vi "pulmonarytesting.vi"() -> ()   [LabVIEW 2014]
uses:
  <vilib>/vision/NI_Vision_Development_Module.lvlib
  <instrlib>/KD Scientific 2XX Series/KD Scientific 2XX Series.lvlib
panel:
  in  "Baud Rate (9600)":u32(ring)=9600 items=["300"=300, "1200"=1200, "2400"=2400, "4800"=4800, "9600"=9600]
  in  "Withdrawal Settings":T1={"Flow Rate (5)"=5.0, "Volume (10)"=10.0, "Volume Units (ml)"=enum."milliliters (ml)", "Rate Units (ml/min.)"=enum."milliliters per minute (ml/min.)"} {"Volume (10)" format="%#.3g"}
  in  "Diameter (8.75 mm)":dbl=8.75
  in  "Infusion Settings":T1={"Flow Rate (5)"=5.0, "Volume (10)"=10.0, "Volume Units (ml)"=enum."milliliters (ml)", "Rate Units (ml/min.)"=enum."milliliters per minute (ml/min.)"}
  out "Status":T2
  in  "stop 2":bool
  out "Delivered Volume":dbl
  out "Units":string
  in  "Operation Mode (Infuse)":u16(ring) items=["Infuse", "Withdraw", "Infuse-Withdraw", "Withdraw-Infuse", "Continuous"]
  in  "Address (0)":i32 format="%0.0f"
  in  "error in (no error)":errorcluster
  in  "VISA resource name":refnum<visa-resource-name>="COM1"
  in  "stop":bool
  out "Image":T3(plugin-control)
  out "Particle Measurements (Pixels) (Particle Analysis 1)":dbl[][](array[numeric]) format="%.2f"
  out "subarray":dbl[](array[numeric])
  out "The diameter":dbl[](array[numeric])
  out "Image from  Vision Acquisition 1":T3(plugin-control)
  in  "stop (F)":bool
  out "Data from Transducer":dynamicdata(graph) caption="Voltage from Transducer V"
  out "Voltage from pressure transducer":dbl[](array[numeric])
  out "Pressure mm Hg":dbl[](graph)
  in  "Calibration factor":dbl[](array[numeric])
  in  "Zero Error":dbl[](array[numeric])
  out "pressure mm Hg":dbl[](array[numeric])
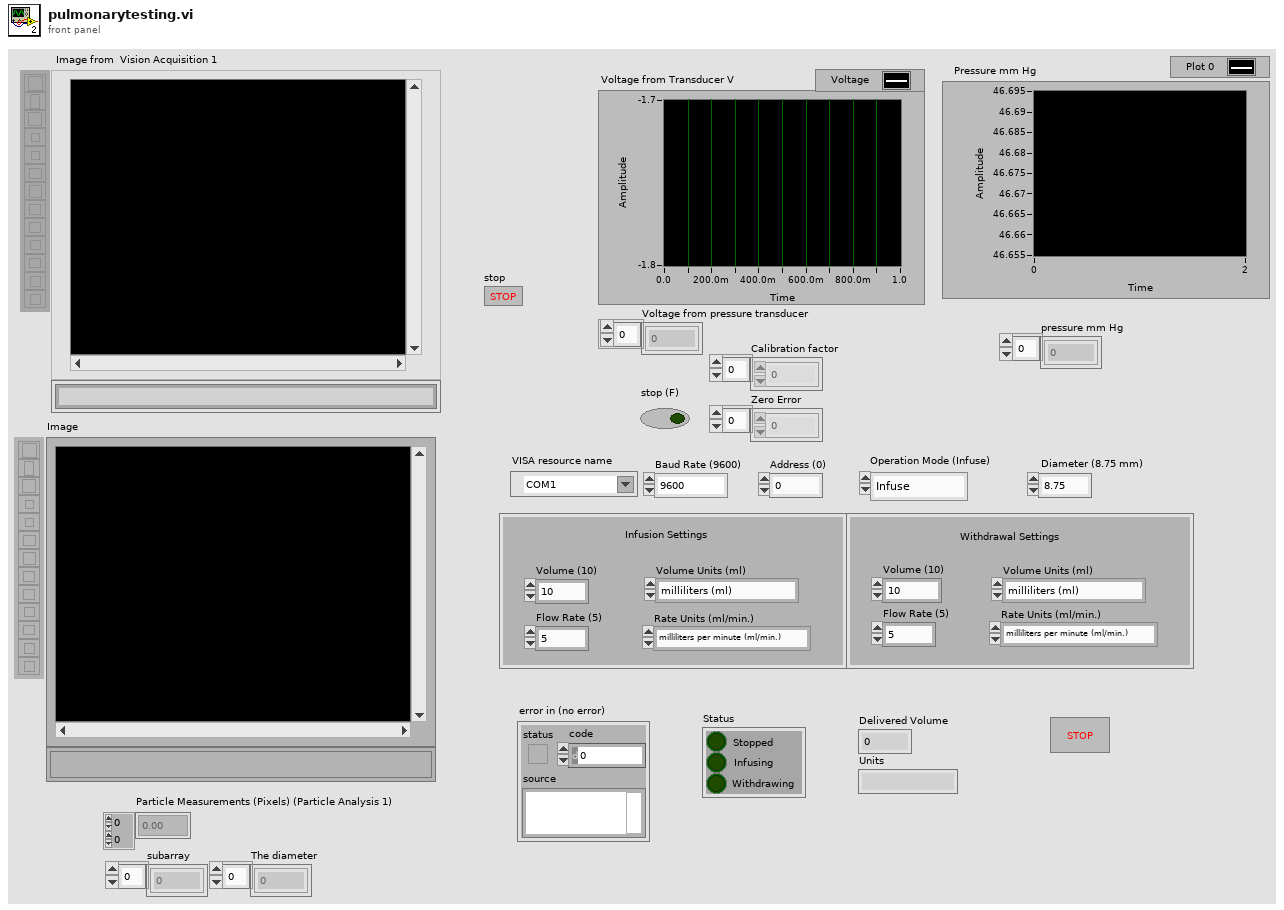
[diagram p1: front panel]
types:
  T1 = cluster{"Flow Rate (5)":dbl, "Volume (10)":dbl, "Volume Units (ml)":enum16{"milliliters (ml)", "microliters (ul)"}, "Rate Units (ml/min.)":enum16{"milliliters per minute (ml/min.)", "milliliters per hour (ml/hr.)", "microliters per minute (ul/min.)", "microliters per hour (ul/hr.)"}}
  T2 = cluster{"Stopped":bool, "Infusing":bool, "Withdrawing":bool}
  T3 = typedef "IMAQ Image.ctl" = refnum<image>
  T4 = typedef "Board Id" = u8
  T5 = typedef "ROI Descriptor" = cluster{"Global Rectangle":i32[], "Contours":cluster{"ID":enum32{"External", "Internal"}, "Type":u32, "Coordinates":i32[]}[]}
  T6 = enum16{"milliliters per minute (ml/min.)", "milliliters per hour (ml/hr.)", "microliters per minute (ul/min.)", "microliters per hour (ul/hr.)"}
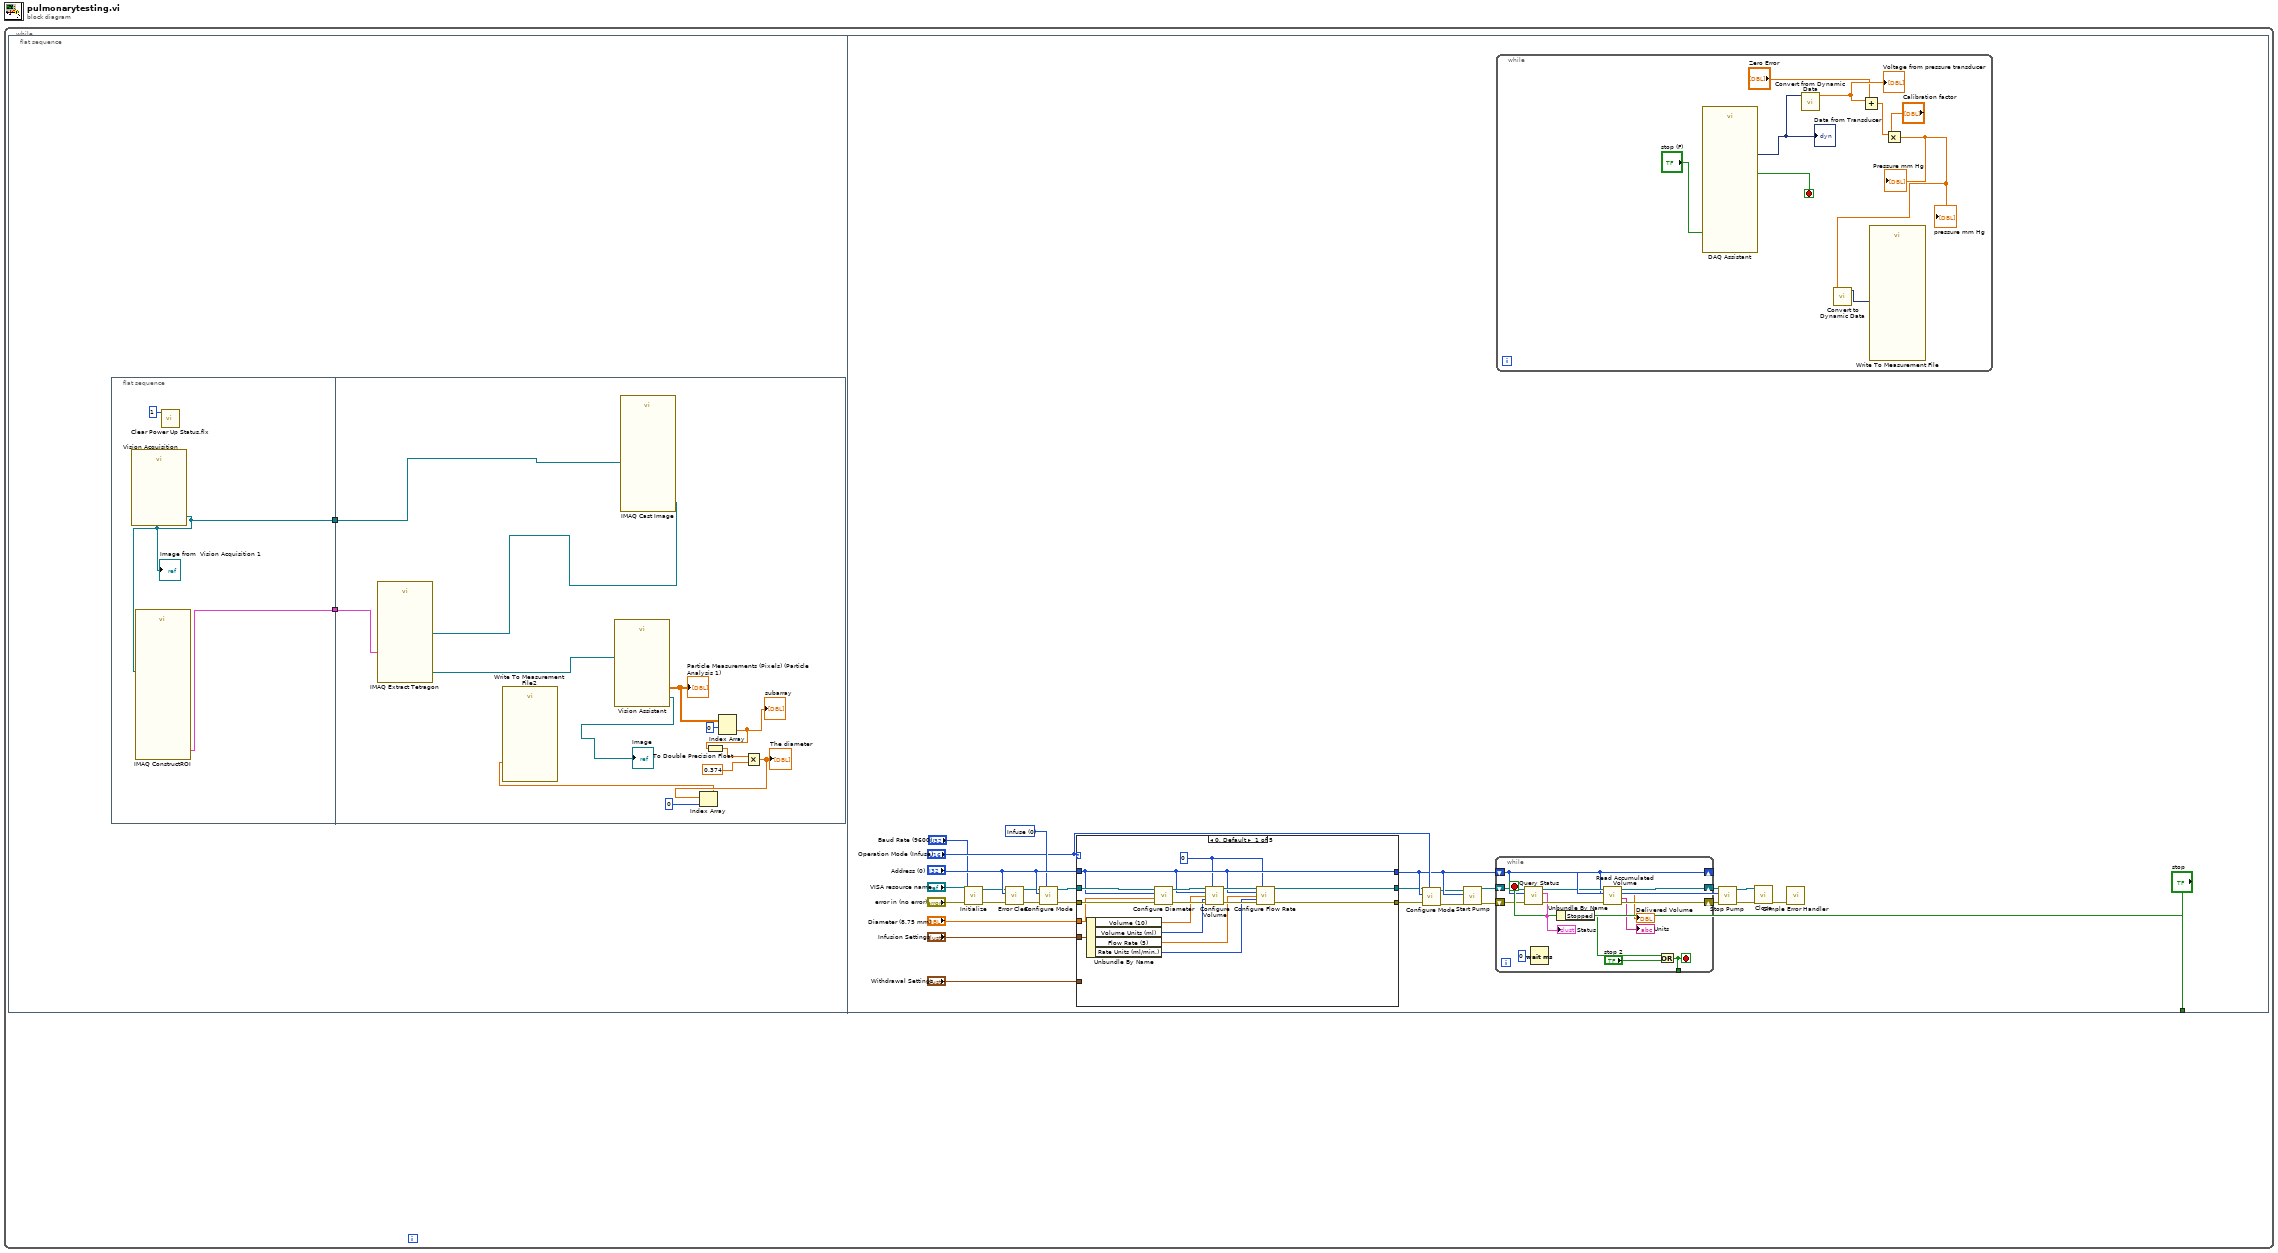
[diagram p0: block diagram]
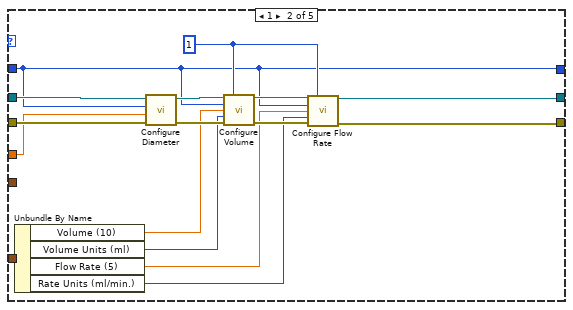
[diagram p2: hidden frame]
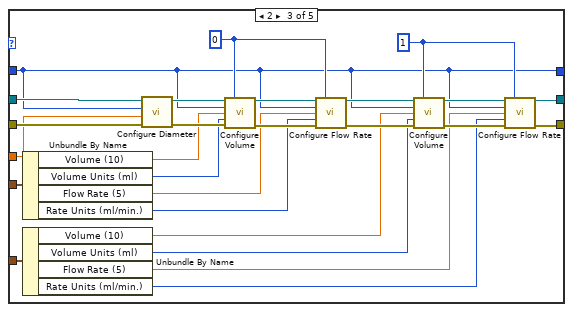
[diagram p3: hidden frame]
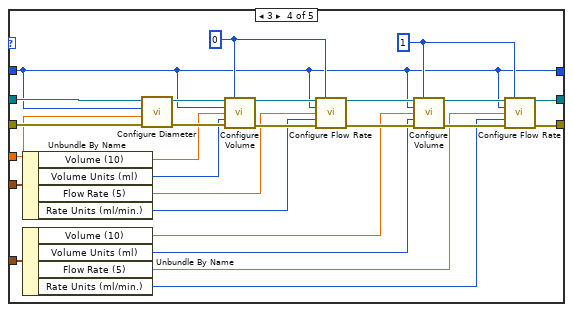
[diagram p4: hidden frame]
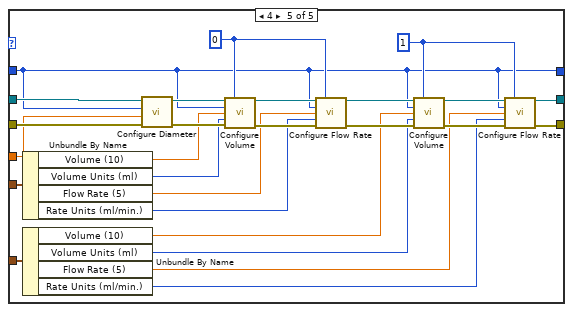
[diagram p5: hidden frame]
diagram:
  n1 = while {
    stop <- w1 stop-if-true
    n2 = flat-sequence {
      tunnel: ["stop"] -> w1
      frame #0 {
        n3 = flat-sequence {
          tunnel: [w6] -> w3
          tunnel: [w4] -> w2
          tunnel: w3 -> [w19]
          tunnel: w2 -> [w10]
          frame #0 {
            n4 = call "Vision Acquisition"() -> ("Image Out"=w4:T3)  [unwired: 25 in, 2 out]
            "Image from  Vision Acquisition 1" <- w4
            n5 = call "IMAQ ConstructROI"("Image"=w4) -> ("ROI Descriptor Out"=w6:T5)  [unwired: 7 in, 3 out]
            n6 = call <vilib>:"Clear Power Up Status.flx"("Board ID"=T4 1) -> ()  [unwired: 6 in, 2 out]
          }
          frame #1 {
            n7 = call "IMAQ Cast Image"("Image Src"=w10) -> ("Image Dst Out"=w16:T3)  [unwired: 9 in, 1 out]
            n8 = call-poly "IMAQ Extract Tetragon"("ROI Descriptor"=w19, "Image Src"=w16) -> ("Image Dst Out"=w17:T3)  [unwired: 8 in, 1 out]
            n9 = call "Vision Assistant"("Image In"=w17) -> ("Image Out"=→"Image":T3, "Particle Measurements (Pixels) (Particle Analysis 1)"=w15:dbl[][])  [unwired: 23 in, 2 out]
            "Particle Measurements (Pixels) (Particle Analysis 1)" <- w15
            n10 = Index Array(array=w15, index (row)=0) -> (element=w13:dbl[])  [unwired: 1 in]
            "subarray" <- w13
            n11 = To Double Precision Float(number=w13) -> (double precision float=w12:dbl[])
            n12 = Multiply(x=w12, y=0.374) -> (x*y=w9:dbl[])
            "The diameter" <- w9
            n13 = Index Array(array=w9, index=0) -> (element=w7:dbl)
            n14 = call "Write To Measurement File2"("Signals"=w7) -> ()  [unwired: 16 in, 3 out]
          }
        }
      }
      frame #1 {
        w42 = u16 0 items=["Infuse", "Withdraw", "Infuse-Withdraw", "Withdraw-Infuse", "Continuous"] ("Mode (infuse)")
        n15 = call <instrlib>:"Initialize.vi"("error in (no error)"="error in (no error)", "Baud Rate (9600)"="Baud Rate (9600)", "VISA resource name"="VISA resource name") -> ("error out"=w45:errorcluster, "VISA resource name out"=w46:refnum<visa-resource-name>)  [unwired: 7 in]
        n16 = call <instrlib>:"Error Clear.vi"("error in (no error)"=w45, "Address (0)"="Address (0)", "VISA resource name"=w46) -> ("error out"=w44:errorcluster, "VISA resource name out"=w43:refnum<visa-resource-name>)  [unwired: 6 in, 1 out]
        n17 = call <instrlib>:"Configure Mode.vi"("Mode (infuse)"=w42, "error in (no error)"=w44, "Address (0)"="Address (0)", "VISA resource name"=w43) -> ("error out"=w40:errorcluster, "VISA resource name out"=w41:refnum<visa-resource-name>)  [unwired: 6 in]
        n18 = case shown="0, Default" "Operation Mode (Infuse)" {
          tunnel: "Infusion Settings" -> [w58 _ w106 w132 w158]
          tunnel: "Withdrawal Settings" -> [_ w80 w105 w131 w157]
          tunnel: w41 -> [w64 w79 w104 w130 w156]
          tunnel: w40 -> [w63 w75 w103 w129 w155]
          tunnel: "Diameter (8.75 mm)" -> [w57 w71 w86 w112 w138]
          tunnel: [w56 w65 w81 w107 w133] -> w38
          tunnel: "Address (0)" -> [w56 w65 w81 w107 w133]
          tunnel: [w51 w76 w83 w109 w135] -> w34
          tunnel: [w50 w72 w82 w108 w134] -> w35
          frame 0, Default {
            w49 = 0
            n19 = Unbundle By Name(w58) -> ("Volume (10)"=w55:dbl, "Volume Units (ml)"=w54:enum16{"milliliters (ml)", "microliters (ul)"}, "Flow Rate (5)"=w53:dbl, "Rate Units (ml/min.)"=w52:T6)
            n20 = call <instrlib>:"Configure Diameter.vi"("error in (no error)"=w63, "Diameter (8.75 mm)"=w57, "Address (0)"=w56, "VISA resource name"=w64) -> ("error out"=w61:errorcluster, "VISA resource name out"=w62:refnum<visa-resource-name>)  [unwired: 6 in]
            n21 = call <instrlib>:"Configure Volume.vi"("VISA resource name"=w62, "Mode (infuse)"=w49, "Address (0)"=w56, "Volume (100)"=w55, "Units (0: milliliters)"=w54, "error in (no error)"=w61) -> ("VISA resource name out"=w60:refnum<visa-resource-name>, "error out"=w59:errorcluster)  [unwired: 8 in]
            n22 = call <instrlib>:"Configure Flow Rate.vi"("VISA resource name"=w60, "Mode (infuse)"=w49, "Address (0)"=w56, "Flow Rate (5)"=w53, "Units (0: milliliters per minute)"=w52, "error in (no error)"=w59) -> ("VISA resource name out"=w51:refnum<visa-resource-name>, "error out"=w50:errorcluster)  [unwired: 8 in]
          }
          frame 1 {
            w66 = 1
            n23 = Unbundle By Name(w80) -> ("Volume (10)"=w70:dbl, "Volume Units (ml)"=w69:enum16{"milliliters (ml)", "microliters (ul)"}, "Flow Rate (5)"=w68:dbl, "Rate Units (ml/min.)"=w67:T6)
            n24 = call <instrlib>:"Configure Diameter.vi"("error in (no error)"=w75, "Diameter (8.75 mm)"=w71, "Address (0)"=w65, "VISA resource name"=w79) -> ("error out"=w74:errorcluster, "VISA resource name out"=w78:refnum<visa-resource-name>)  [unwired: 6 in]
            n25 = call <instrlib>:"Configure Volume.vi"("VISA resource name"=w78, "Mode (infuse)"=w66, "Address (0)"=w65, "Volume (100)"=w70, "Units (0: milliliters)"=w69, "error in (no error)"=w74) -> ("VISA resource name out"=w77:refnum<visa-resource-name>, "error out"=w73:errorcluster)  [unwired: 8 in]
            n26 = call <instrlib>:"Configure Flow Rate.vi"("VISA resource name"=w77, "Mode (infuse)"=w66, "Address (0)"=w65, "Flow Rate (5)"=w68, "Units (0: milliliters per minute)"=w67, "error in (no error)"=w73) -> ("VISA resource name out"=w76:refnum<visa-resource-name>, "error out"=w72:errorcluster)  [unwired: 8 in]
          }
          frame 2 {
            w84 = 1
            w85 = 0
            n27 = Unbundle By Name(w106) -> ("Volume (10)"=w94:dbl, "Volume Units (ml)"=w93:enum16{"milliliters (ml)", "microliters (ul)"}, "Flow Rate (5)"=w92:dbl, "Rate Units (ml/min.)"=w91:T6)
            n28 = Unbundle By Name(w105) -> ("Volume (10)"=w90:dbl, "Volume Units (ml)"=w89:enum16{"milliliters (ml)", "microliters (ul)"}, "Flow Rate (5)"=w88:dbl, "Rate Units (ml/min.)"=w87:T6)
            n29 = call <instrlib>:"Configure Diameter.vi"("error in (no error)"=w103, "Diameter (8.75 mm)"=w86, "Address (0)"=w81, "VISA resource name"=w104) -> ("error out"=w98:errorcluster, "VISA resource name out"=w102:refnum<visa-resource-name>)  [unwired: 6 in]
            n30 = call <instrlib>:"Configure Volume.vi"("VISA resource name"=w102, "Mode (infuse)"=w85, "Address (0)"=w81, "Volume (100)"=w94, "Units (0: milliliters)"=w93, "error in (no error)"=w98) -> ("VISA resource name out"=w101:refnum<visa-resource-name>, "error out"=w97:errorcluster)  [unwired: 8 in]
            n31 = call <instrlib>:"Configure Flow Rate.vi"("VISA resource name"=w101, "Mode (infuse)"=w85, "Address (0)"=w81, "Flow Rate (5)"=w92, "Units (0: milliliters per minute)"=w91, "error in (no error)"=w97) -> ("VISA resource name out"=w100:refnum<visa-resource-name>, "error out"=w96:errorcluster)  [unwired: 8 in]
            n32 = call <instrlib>:"Configure Volume.vi"("VISA resource name"=w100, "Mode (infuse)"=w84, "Address (0)"=w81, "Volume (100)"=w90, "Units (0: milliliters)"=w89, "error in (no error)"=w96) -> ("VISA resource name out"=w99:refnum<visa-resource-name>, "error out"=w95:errorcluster)  [unwired: 8 in]
            n33 = call <instrlib>:"Configure Flow Rate.vi"("VISA resource name"=w99, "Mode (infuse)"=w84, "Address (0)"=w81, "Flow Rate (5)"=w88, "Units (0: milliliters per minute)"=w87, "error in (no error)"=w95) -> ("VISA resource name out"=w83:refnum<visa-resource-name>, "error out"=w82:errorcluster)  [unwired: 8 in]
          }
          frame 3 {
            w110 = 1
            w111 = 0
            n34 = Unbundle By Name(w132) -> ("Volume (10)"=w120:dbl, "Volume Units (ml)"=w119:enum16{"milliliters (ml)", "microliters (ul)"}, "Flow Rate (5)"=w118:dbl, "Rate Units (ml/min.)"=w117:T6)
            n35 = Unbundle By Name(w131) -> ("Volume (10)"=w116:dbl, "Volume Units (ml)"=w115:enum16{"milliliters (ml)", "microliters (ul)"}, "Flow Rate (5)"=w114:dbl, "Rate Units (ml/min.)"=w113:T6)
            n36 = call <instrlib>:"Configure Diameter.vi"("error in (no error)"=w129, "Diameter (8.75 mm)"=w112, "Address (0)"=w107, "VISA resource name"=w130) -> ("error out"=w124:errorcluster, "VISA resource name out"=w128:refnum<visa-resource-name>)  [unwired: 6 in]
            n37 = call <instrlib>:"Configure Volume.vi"("VISA resource name"=w128, "Mode (infuse)"=w111, "Address (0)"=w107, "Volume (100)"=w120, "Units (0: milliliters)"=w119, "error in (no error)"=w124) -> ("VISA resource name out"=w127:refnum<visa-resource-name>, "error out"=w123:errorcluster)  [unwired: 8 in]
            n38 = call <instrlib>:"Configure Flow Rate.vi"("VISA resource name"=w127, "Mode (infuse)"=w111, "Address (0)"=w107, "Flow Rate (5)"=w118, "Units (0: milliliters per minute)"=w117, "error in (no error)"=w123) -> ("VISA resource name out"=w126:refnum<visa-resource-name>, "error out"=w122:errorcluster)  [unwired: 8 in]
            n39 = call <instrlib>:"Configure Volume.vi"("VISA resource name"=w126, "Mode (infuse)"=w110, "Address (0)"=w107, "Volume (100)"=w116, "Units (0: milliliters)"=w115, "error in (no error)"=w122) -> ("VISA resource name out"=w125:refnum<visa-resource-name>, "error out"=w121:errorcluster)  [unwired: 8 in]
            n40 = call <instrlib>:"Configure Flow Rate.vi"("VISA resource name"=w125, "Mode (infuse)"=w110, "Address (0)"=w107, "Flow Rate (5)"=w114, "Units (0: milliliters per minute)"=w113, "error in (no error)"=w121) -> ("VISA resource name out"=w109:refnum<visa-resource-name>, "error out"=w108:errorcluster)  [unwired: 8 in]
          }
          frame 4 {
            w136 = 1
            w137 = 0
            n41 = Unbundle By Name(w158) -> ("Volume (10)"=w146:dbl, "Volume Units (ml)"=w145:enum16{"milliliters (ml)", "microliters (ul)"}, "Flow Rate (5)"=w144:dbl, "Rate Units (ml/min.)"=w143:T6)
            n42 = Unbundle By Name(w157) -> ("Volume (10)"=w142:dbl, "Volume Units (ml)"=w141:enum16{"milliliters (ml)", "microliters (ul)"}, "Flow Rate (5)"=w140:dbl, "Rate Units (ml/min.)"=w139:T6)
            n43 = call <instrlib>:"Configure Diameter.vi"("error in (no error)"=w155, "Diameter (8.75 mm)"=w138, "Address (0)"=w133, "VISA resource name"=w156) -> ("error out"=w150:errorcluster, "VISA resource name out"=w154:refnum<visa-resource-name>)  [unwired: 6 in]
            n44 = call <instrlib>:"Configure Volume.vi"("VISA resource name"=w154, "Mode (infuse)"=w137, "Address (0)"=w133, "Volume (100)"=w146, "Units (0: milliliters)"=w145, "error in (no error)"=w150) -> ("VISA resource name out"=w153:refnum<visa-resource-name>, "error out"=w149:errorcluster)  [unwired: 8 in]
            n45 = call <instrlib>:"Configure Flow Rate.vi"("VISA resource name"=w153, "Mode (infuse)"=w137, "Address (0)"=w133, "Flow Rate (5)"=w144, "Units (0: milliliters per minute)"=w143, "error in (no error)"=w149) -> ("VISA resource name out"=w152:refnum<visa-resource-name>, "error out"=w148:errorcluster)  [unwired: 8 in]
            n46 = call <instrlib>:"Configure Volume.vi"("VISA resource name"=w152, "Mode (infuse)"=w136, "Address (0)"=w133, "Volume (100)"=w142, "Units (0: milliliters)"=w141, "error in (no error)"=w148) -> ("VISA resource name out"=w151:refnum<visa-resource-name>, "error out"=w147:errorcluster)  [unwired: 8 in]
            n47 = call <instrlib>:"Configure Flow Rate.vi"("VISA resource name"=w151, "Mode (infuse)"=w136, "Address (0)"=w133, "Flow Rate (5)"=w140, "Units (0: milliliters per minute)"=w139, "error in (no error)"=w147) -> ("VISA resource name out"=w135:refnum<visa-resource-name>, "error out"=w134:errorcluster)  [unwired: 8 in]
          }
        }
        n48 = call <instrlib>:"Configure Mode.vi"("Mode (infuse)"="Operation Mode (Infuse)", "error in (no error)"=w35, "Address (0)"=w38, "VISA resource name"=w34) -> ("error out"=w37:errorcluster, "VISA resource name out"=w36:refnum<visa-resource-name>)  [unwired: 6 in]
        n49 = call <instrlib>:"Start Pump.vi"("error in (no error)"=w37, "Address (0)"=w38, "VISA resource name"=w36) -> ("error out"=w23:errorcluster, "VISA resource name out"=w22:refnum<visa-resource-name>)  [unwired: 7 in]
        n50 = while {
          shift-right: [w162] -> w29
          shift-left: w38 -> [w162]
          shift-right: [w164] -> w24
          shift-left: w22 -> [w169]
          shift-right: [w163] -> w25
          shift-left: w23 -> [w170]
          tunnel: [w159] -> _
          stop <- w159 stop-if-true
          n51 = call <instrlib>:"Query Status.vi"("error in (no error)"=w170, "Address (0)"=w162, "VISA resource name"=w169) -> ("error out"=w172:errorcluster, "Status"=w168:T2, "VISA resource name out"=w165:refnum<visa-resource-name>)  [unwired: 6 in]
          "Status" <- w168
          n52 = Wait (ms)(milliseconds to wait=u32 0) -> ()  [unwired: 1 out]
          n53 = Unbundle By Name(w168) -> ("Stopped"=w167:bool)
          n54 = call <instrlib>:"Read Accumulated Volume.vi"("error in (no error)"=w172, "Address (0)"=w162, "VISA resource name"=w165) -> ("error out"=w163:errorcluster, "Units"=→"Units":string, "Delivered Volume"=→"Delivered Volume":dbl, "VISA resource name out"=w164:refnum<visa-resource-name>)  [unwired: 5 in]
          n55 = Or(x=w167, y="stop 2") -> (x .or. y?=w159:bool)
        }
        n56 = while {
          stop <- w180 stop-if-true
          n57 = call "DAQ Assistant"("stop (F)"="stop (F)") -> ("data"=w175:dynamicdata, "stopped"=w180:bool)  [unwired: 15 in, 2 out]
          "Data from Transducer" <- w175
          n58 = call "Convert from Dynamic Data"("Dynamic Data Type"=w175) -> ("Array"=w178:dbl[])  [unwired: 3 in]
          "Voltage from pressure transducer" <- w178
          n59 = Add(x=w178, y="Zero Error") -> (x+y=w176:dbl[])
          n60 = Multiply(x=w176, y="Calibration factor") -> (x*y=w174:dbl[])
          "Pressure mm Hg" <- w174
          "pressure mm Hg" <- w174
          n61 = call "Convert to Dynamic Data"("Array"=w174) -> ("Dynamic Data Type"=w173:dynamicdata)  [unwired: 3 in]
          n62 = call "Write To Measurement File"("Signals"=w173) -> ()  [unwired: 16 in, 3 out]
        }
        n63 = call <instrlib>:"Stop Pump.vi"("error in (no error)"=w25, "Address (0)"=w29, "VISA resource name"=w24) -> ("error out"=w31:errorcluster, "VISA resource name out"=w32:refnum<visa-resource-name>)  [unwired: 7 in]
        n64 = call <instrlib>:"Close.vi"("error in (no error)"=w31, "VISA resource name"=w32) -> ("error out"=w30:errorcluster)  [unwired: 9 in]
        n65 = call <vilib>:"Simple Error Handler.vi"("error in (no error)"=w30) -> ()  [unwired: 4 in, 5 out]
      }
    }
  }
